vi "Write VI Reference.vi"(8 "error in (no error)":errorcluster, 10 "VI Reference Wrappers":cluster{"VI Refnum":refnum<vi>, "Name":string}[](array[cluster]), 11 "UI Reference Wrapper in":refnum<class "UI Reference Wrapper.lvclass">) -> (0 "error out":errorcluster, 3 "UI Reference Wrapper out":refnum<class "UI Reference Wrapper.lvclass">)   [LabVIEW 2015, in "UI Reference Wrapper.lvclass"]
uses:
  UI Reference Wrapper.lvclass
  UI Reference Wrapper.lvclass/UI Reference Wrapper.ctl
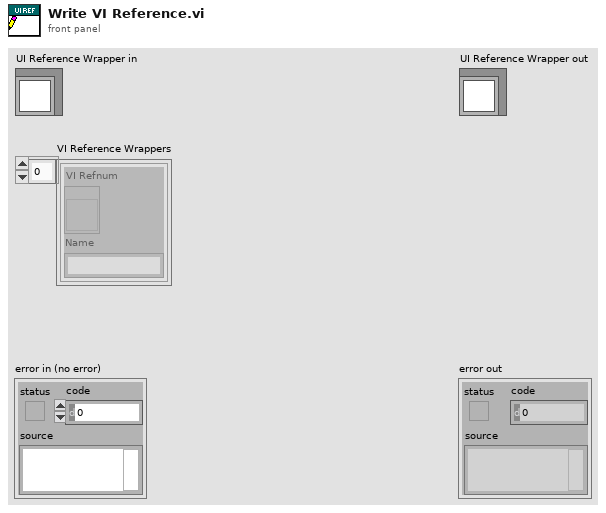
[diagram p1: front panel]
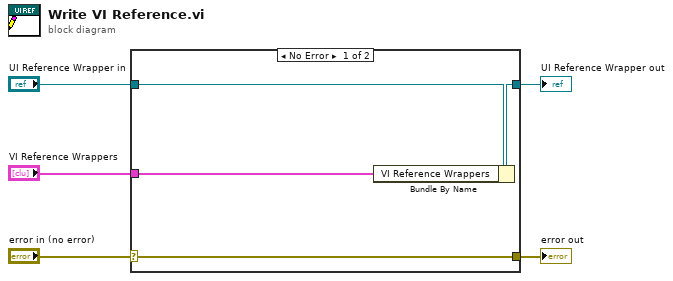
[diagram p0: block diagram]
diagram:
  n1 = case shown="No Error" "error in (no error)" {
    selector: "error in (no error)" -> [w9 w10]
    tunnel: [w9 w10] -> w4
    tunnel: [w7 w11] -> w2
    tunnel: "UI Reference Wrapper in" -> [w8 w11]
    tunnel: "VI Reference Wrappers" -> [w6 _]
    frame No Error {
      n2 = Bundle By Name(cluster=w8, "VI Reference Wrappers"=w6) -> (w7:refnum<class "UI Reference Wrapper.lvclass">)
    }
    frame Error {
    }
  }
  "error out" <- w4
  "UI Reference Wrapper out" <- w2
